vi "CRYInsert All.vi"(4 "Waves":T1 {"Y dB ref" format="%.1f"; "Y axis" items=["Log", "Lin"]; "Y data" items=["dB", "Lin"]; "X data" items=["dB", "Lin"]}, 6 "Results":T3 {"Margin" format="%.2f"}, 7 "sOption2":string, 8 "sOption1":string, 9 "Curves":T5 {"Z data" items=["dB", "Lin"]; "X data" items=["dB", "Lin"]; "Y data" items=["dB", "Lin"]; "Z dB ref" format="%.1f"; "Z axis" items=["Log", "Lin"]; "X dB ref" format="%.1f"; "X axis" items=["Log", "Lin"]; "Y axis" items=["Log", "Lin"]; "Y dB ref" format="%.1f"; "Curve"."z" format="%.2f"; "Curve"."y" format="%.2f"; "Curve"."x" format="%.2f"}, 10 "Step No.":i32, 11 "Type In":enum16{"Curves", "Values", "Results", "WFM"}(ring)) -> (2 "Inserted Names Out":string[](array[string]), 3 "Type Out":enum16{"Curves", "Values", "Results", "WFM"}(ring))   [LabVIEW 2013]
uses:
  CRYSystem/Typedef Control/CRYData Cluster Array.ctl
  CRYSystem/Typedef Control/CRYData Cluster.ctl
  CRYSystem/Typedef Control/CRYResult Cluster Array.ctl
  CRYSystem/Typedef Control/CRYResult Cluster.ctl
  CRYSystem/Typedef Control/CRYWaveform Cluster Array.ctl
  CRYSystem/Typedef Control/CRYWaveform Cluster.ctl
  Global/CRYCurve Library Global.vi
  CRYSystem/Task Sequence/CRYProject Run Control Global.vi
panel:
  out "wav2":i32[](array[numeric])
  out "wav1":i32[](array[numeric])
  out "res2":i32[](array[numeric])
  out "res1":i32[](array[numeric])
  out "val1":i32[](array[numeric])
  out "val2":i32[](array[numeric])
  out "cur1":i32[](array[numeric])
  out "cur2":i32[](array[numeric])
  out "x-y":i32[](array[numeric])
  out "Type":string[](array[string])
  out "Deleted Names":string[](array[string])
  out "Inserted Names":string[](array[string])
  out "Inserted Index":i32[](array[numeric])
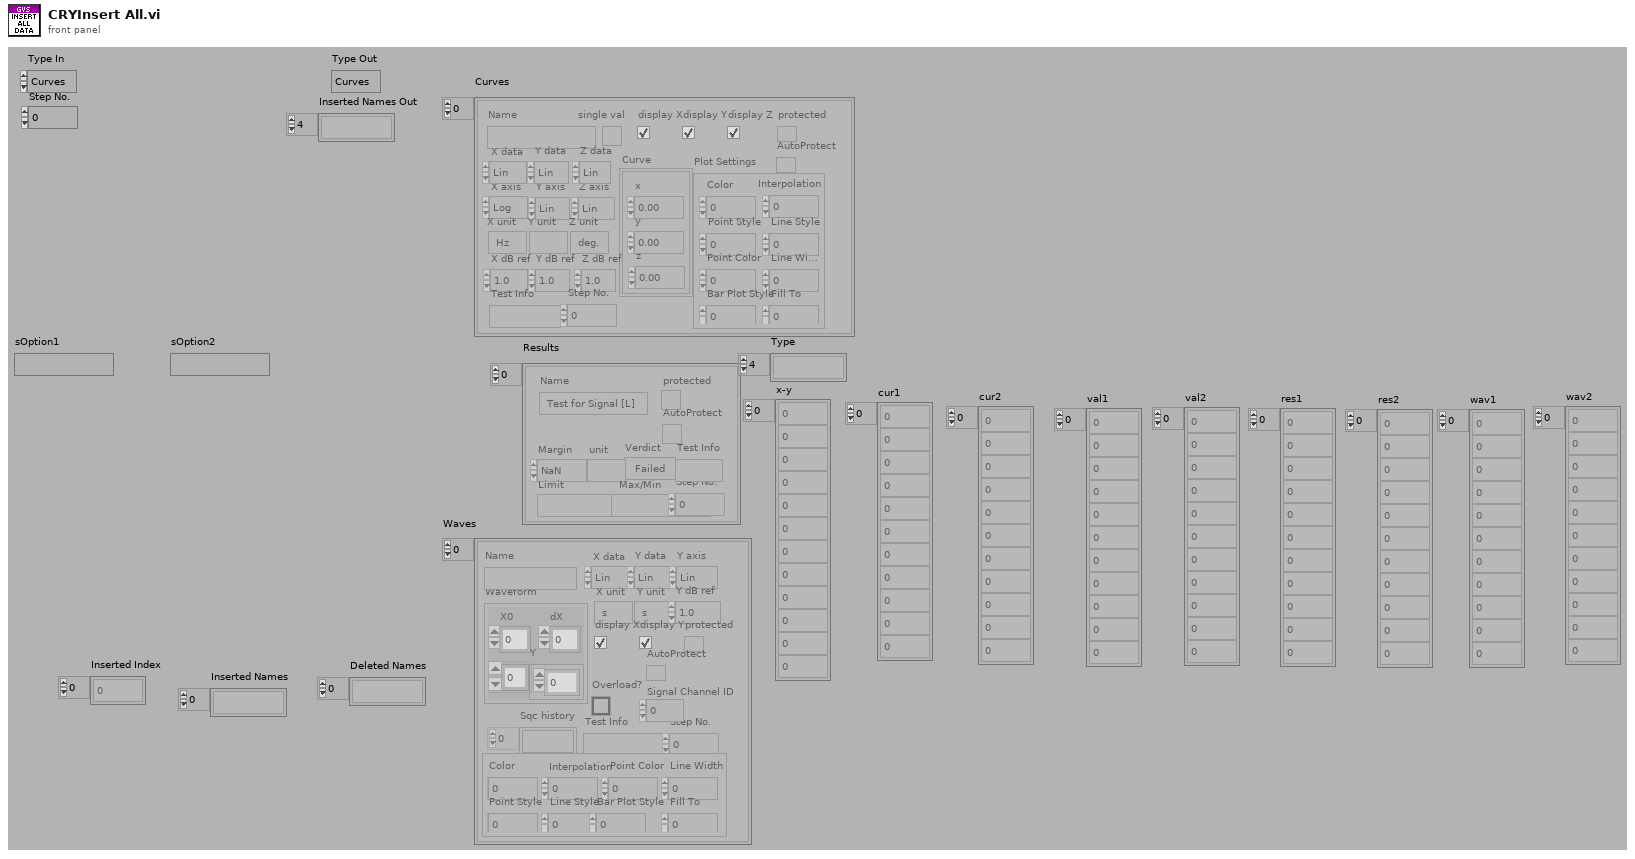
[diagram p1: front panel]
types:
  T1 = typedef "CRYWaveform Cluster Array.ctl" = T2[]
  T2 = typedef "CRYWaveform Cluster.ctl" = cluster{"Waveform":cluster{"X0":dbl, "dX":dbl, "Y":sgl[]}, "X data":u16, "Y data":u16, "Y axis":u16, "X unit":string, "Y unit":string, "Y dB ref":dbl, "display Y":bool, "display X":bool, "Overload?":bool, "Test Info":string, "Step No.":i32, "Name":string, "protected":bool, "Sqc history":string[], "Signal Channel ID":i32, "Plot Settings":cluster{"Color":u32, "Interpolation":u8, "Point Style":u8, "Line Style":u8, "Point Color":u32, "Line Width":u8, "Bar Plot Style":u8, "Fill To":i16}, "AutoProtect":bool}
  T3 = typedef "CRYResult Cluster Array.ctl" = T4[]
  T4 = typedef "CRYResult Cluster.ctl" = cluster{"Name":string, "Margin":dbl, "unit":string, "Verdict":bool, "Limit":string, "Max/Min":string, "protected":bool, "Step No.":i32, "Test Info":string, "AutoProtect":bool}
  T5 = typedef "CRYData Cluster Array.ctl" = T6[]
  T6 = typedef "CRYData Cluster.ctl" = cluster{"Name":string, "Curve":cluster{"x":dbl, "y":dbl, "z":dbl}[], "X data":u16, "Y data":u16, "Z data":u16, "X axis":u16, "Y axis":u16, "Z axis":u16, "X unit":string, "Y unit":string, "Z unit":string, "X dB ref":dbl, "Y dB ref":dbl, "Z dB ref":dbl, "single val":bool, "protected":bool, "display X":bool, "display Y":bool, "display Z":bool, "Test Info":string, "Step No.":i32, "Plot Settings":cluster{"Color":u32, "Interpolation":u8, "Point Style":u8, "Line Style":u8, "Point Color":u32, "Line Width":u8, "Bar Plot Style":u8, "Fill To":i16}, "AutoProtect":bool}
  T7 = cluster{"Color":u32, "Interpolation":u8, "Point Style":u8, "Line Style":u8, "Point Color":u32, "Line Width":u8, "Bar Plot Style":u8, "Fill To":i16}
  T8 = cluster{"CurveOld":string[], "ValueOld":string[], "ResultOld":string[], "WFMOld":string[], "CurveNew":string[], "ValueNew":string[], "ResultNew":string[], "WFMNew":string[]}
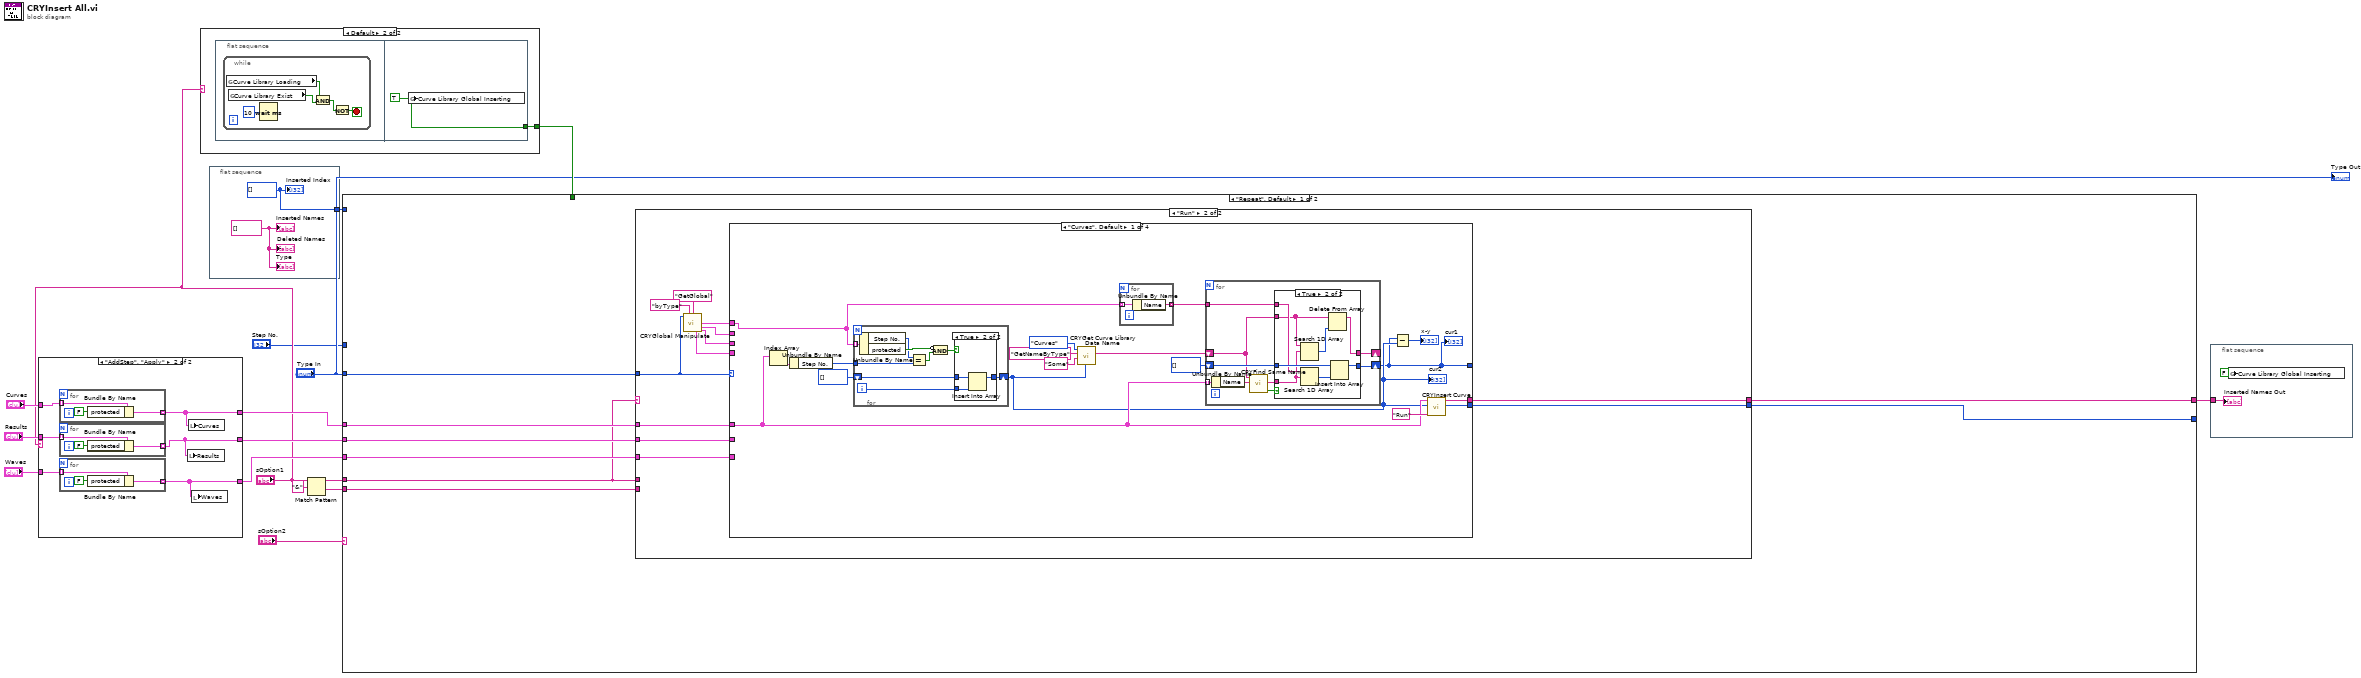
[diagram p0: block diagram]
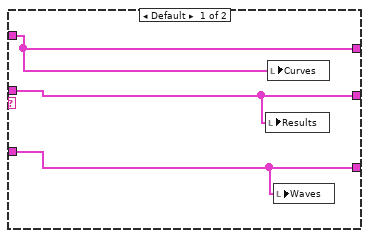
[diagram p2: hidden frame]
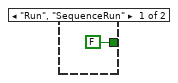
[diagram p3: hidden frame]
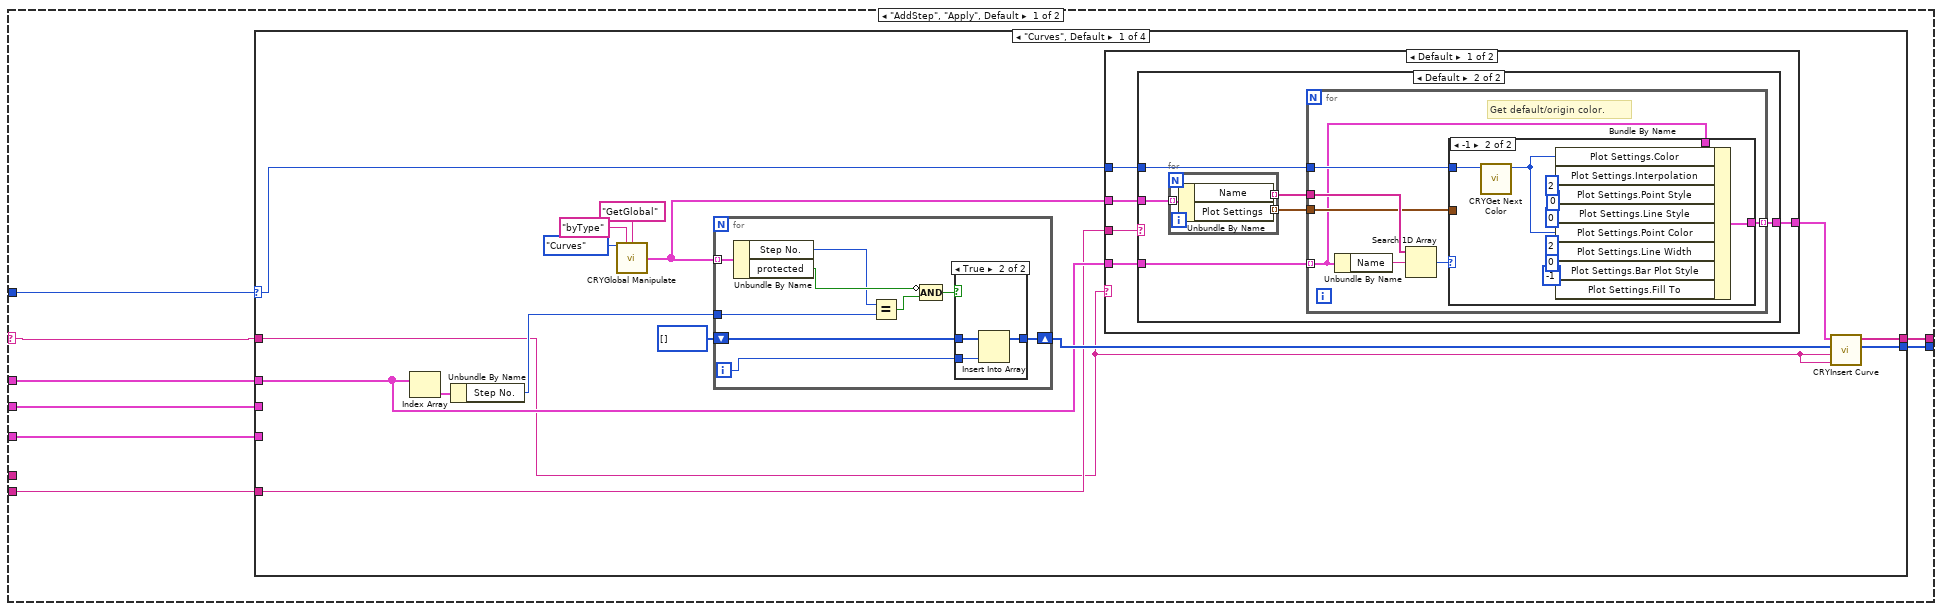
[diagram p4: hidden frame]
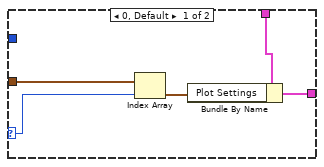
[diagram p7: hidden frame]
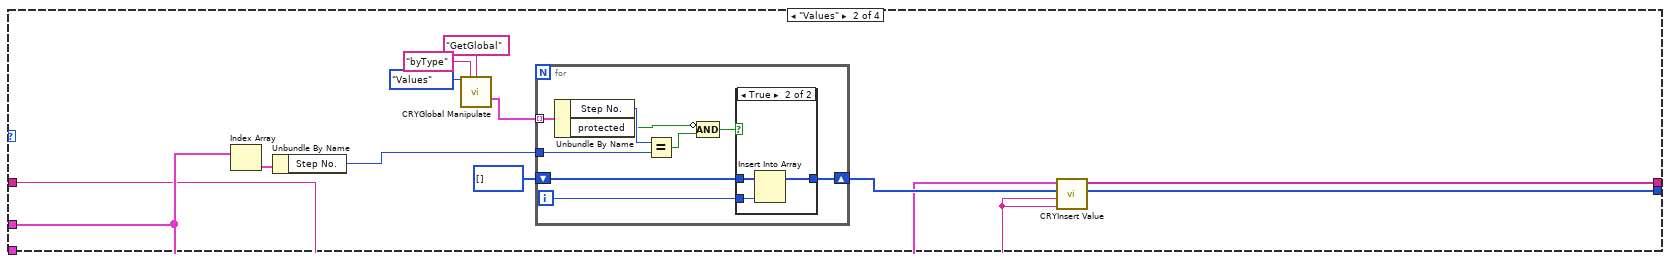
[diagram p9: hidden frame]
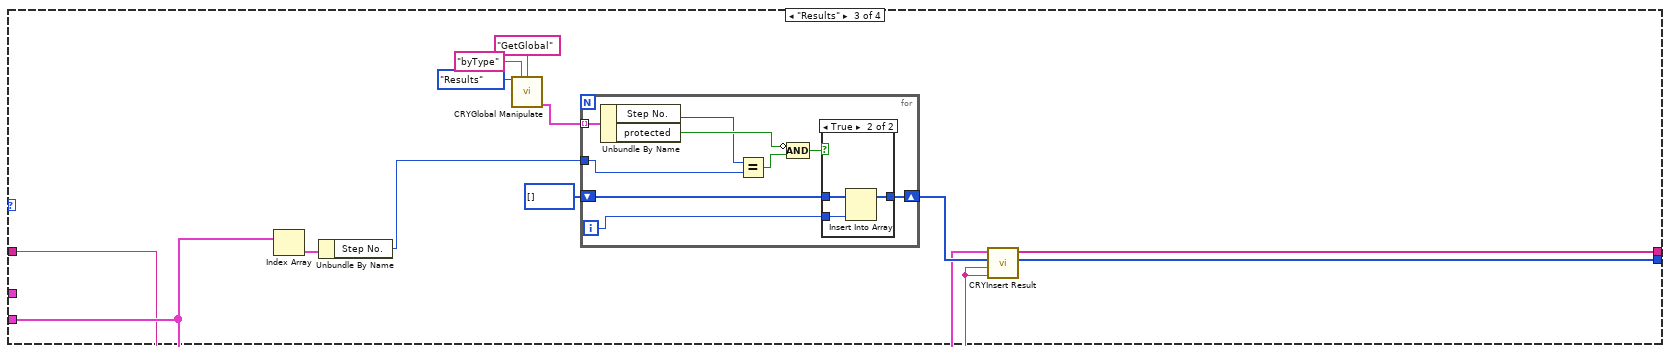
[diagram p11: hidden frame]
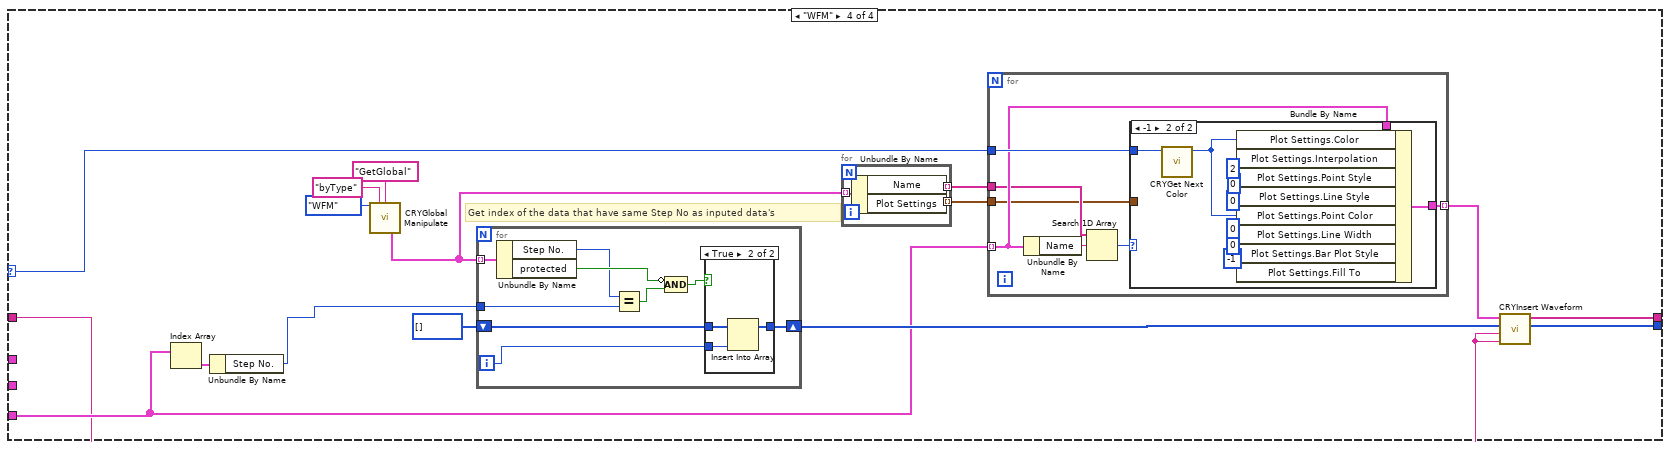
[diagram p13: hidden frame]
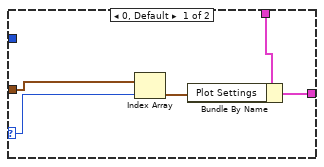
[diagram p14: hidden frame]
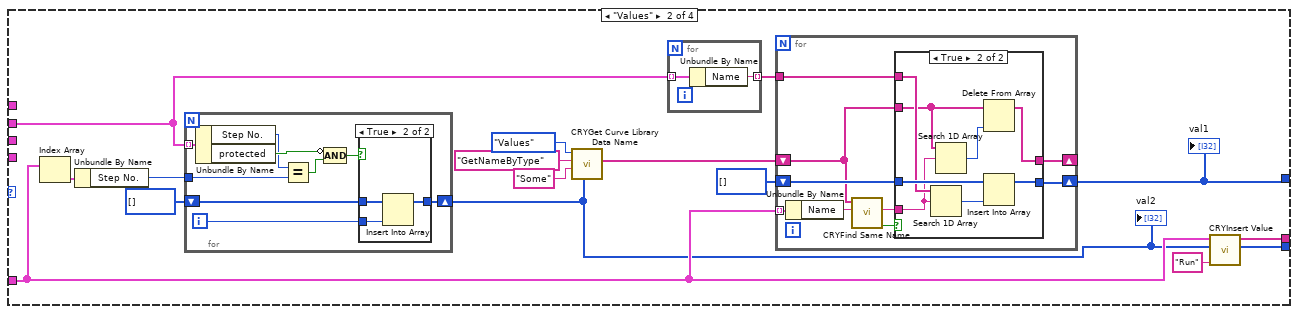
[diagram p18: hidden frame]
diagram:
  n1 = case shown="\"AddStep\", \"Apply\"" "sOption1" {
    tunnel: "Curves" -> [w19 w25]
    tunnel: [w19 w24] -> w7
    tunnel: "Waves" -> [w18 w23]
    tunnel: [w18 w22] -> w5
    tunnel: "Results" -> [w17 w21]
    tunnel: [w17 w20] -> w3
    frame Default {
      n2 = local write "Results"(w17) -> ()
      n3 = local write "Curves"(w19) -> ()
      n4 = local write "Waves"(w18) -> ()
    }
    frame "AddStep", "Apply" {
      n5 = for {
        tunnel: w25 -> [w34] mode=indexing
        tunnel: [w32] -> w24 mode=indexing
        n6 = Bundle By Name(cluster=w34, "protected"=FALSE) -> (w32:T6)
      }
      n7 = for {
        tunnel: w21 -> [w31] mode=indexing
        tunnel: [w29] -> w20 mode=indexing
        n8 = Bundle By Name(cluster=w31, "protected"=FALSE) -> (w29:T4)
      }
      n9 = for {
        tunnel: w23 -> [w28] mode=indexing
        tunnel: [w26] -> w22 mode=indexing
        n10 = Bundle By Name(cluster=w28, "protected"=FALSE) -> (w26:T2)
      }
      n11 = local write "Results"(w20) -> ()
      n12 = local write "Curves"(w24) -> ()
      n13 = local write "Waves"(w22) -> ()
    }
  }
  n14 = case shown="Default" "sOption1" {
    tunnel: [FALSE ("Curve Library Global Inserting") w36] -> w16
    frame "Run", "SequenceRun" {
    }
    frame Default {
      n15 = flat-sequence {
        tunnel: [w42] -> w36
        frame #0 {
          n16 = while {
            stop <- w37 stop-if-true
            n17 = global read "CRYCurve Library Global.vi" "Curve Library Loading"() -> (w39:bool)
            n18 = global read "CRYCurve Library Global.vi" "Curve Library Exist"() -> (w38:bool)
            n19 = Wait (ms)(milliseconds to wait=u32 10) -> ()  [unwired: 1 out]
            n20 = And(x=w39, y=w38) -> (x .and. y?=w40:bool)
            n21 = Not(x=w40) -> (.not. x?=w37:bool)
          }
        }
        frame #1 {
          w42 = TRUE ("Curve Library Global Inserting")
          n22 = global write "CRYCurve Library Global.vi" "Curve Library Global Inserting"(w42) -> ()
        }
      }
    }
  }
  n23 = flat-sequence {
    tunnel: [w44] -> w9
    frame #0 {
      w43 = string[] [] ("Inserted Names")
      w44 = i32[] [] ("Index")
      "Inserted Index" <- w44
      "Inserted Names" <- w43
      "Deleted Names" <- w43
      "Type" <- w43
    }
  }
  n24 = Match Pattern(string="sOption1", regular expression="&") -> (before substring=w13:string, after substring=w12:string)  [unwired: 1 in, 2 out]
  n25 = case shown="\"Repeat\", Default" "sOption2" {
    tunnel: w16 -> [_ _]
    tunnel: [w46 w464] -> w15
    tunnel: [w52 w461] -> _
    tunnel: w7 -> [w49 w465]
    tunnel: "Type In" -> [w45 w463]
    tunnel: w13 -> [w47 _]
    tunnel: w12 -> [w48 _]
    tunnel: w9 -> [_ _]
    tunnel: w3 -> [w51 w453]
    tunnel: w5 -> [w50 w452]
    tunnel: "Step No." -> [_ w444]
    frame "Repeat", Default {
      n26 = case shown="\"Run\"" w47 {
        selector: w47 -> [w53 _]
        tunnel: [w60 w242] -> w46
        tunnel: [w59 w241] -> w52
        tunnel: w45 -> [w54 w235]
        tunnel: w51 -> [w58 w240]
        tunnel: w50 -> [w57 w239]
        tunnel: w49 -> [w56 w238]
        tunnel: w48 -> [w55 _]
        tunnel: w47 -> [_ _]
        frame "AddStep", "Apply", Default {
          n27 = case shown="\"Curves\", Default" w54 {
            selector: w54 -> [w66 _ _ w182]
            tunnel: w56 -> [w73 w135 _ _]
            tunnel: [w75 w138 w163 w192] -> w60
            tunnel: [w71 w136 w160 w188] -> w59
            tunnel: w55 -> [w70 _ _ _]
            tunnel: w58 -> [_ _ w161 _]
            tunnel: w57 -> [_ _ _ w190]
            tunnel: w53 -> [w61 w127 w152 w177]
            frame "Curves", Default {
              n28 = Index Array(array=w73) -> (element=w67:T6)  [unwired: 1 in]
              n29 = Unbundle By Name(w67) -> ("Step No."=w68:i32)
              n30 = call "CRYGlobal Manipulate.vi"("Type"=enum16{"Curves", "Values", "Results", "WFM"}."Curves", "sOption"="byType", "sAction"="GetGlobal") -> ("Curves Out"=w62:T6[])  [unwired: 6 in, 6 out]
              n31 = for {
                tunnel: w68 -> [w76]
                tunnel: w62 -> [w82] mode=indexing
                shift-right: [w83] -> w74
                shift-left: i32[] [] ("Index") -> [w84]
                i -> [w81]
                n32 = Unbundle By Name(w82) -> ("Step No."=w77:i32, "protected"=w78:bool)
                n33 = Equal?(x=w77, y=w76) -> (x = y?=w80:bool)
                n34 = Compound Arithmetic op=AND(invert w78, w80) -> (w79:bool)
                n35 = case shown="True" w79 {
                  tunnel: [w85 w87] -> w83
                  tunnel: w84 -> [w85 w88]
                  tunnel: w81 -> [_ w86]
                  frame False {
                  }
                  frame True {
                    n36 = Insert Into Array(array=w88, new element=w86) -> (w87:i32[])  [unwired: 1 in]
                  }
                }
              }
              n37 = case shown="Default" w61 {
                tunnel: w66 -> [w93 _]
                tunnel: w73 -> [w92 w126]
                tunnel: [w91 w126] -> w72
                tunnel: w70 -> [w90 _]
                tunnel: w62 -> [w89 _]
                frame Default {
                  n38 = case shown="Default" w90 {
                    tunnel: w93 -> [_ w100]
                    tunnel: w92 -> [w94 w99]
                    tunnel: [w94 w98] -> w91
                    tunnel: w89 -> [_ w97]
                    frame "UsePlot" {
                    }
                    frame Default {
                      n39 = for {
                        tunnel: w97 -> [w103] mode=indexing
                        tunnel: [w102] -> w96 mode=indexing
                        tunnel: [w101] -> w95 mode=indexing
                        n40 = Unbundle By Name(w103) -> ("Name"=w102:string, "Plot Settings"=w101:T7)
                      }
                      n41 = for {
                        tunnel: w99 -> [w104] mode=indexing
                        tunnel: [w109] -> w98 mode=indexing
                        tunnel: w100 -> [w110]
                        tunnel: w96 -> [w108]
                        tunnel: w95 -> [w105]
                        # "Get default/origin color."
                        n42 = Unbundle By Name(w104) -> ("Name"=w107:string)
                        n43 = Search 1D Array(1D array=w108, element=w107) -> (index of element=w106:i32)  [unwired: 1 out]
                        n44 = case shown="-1" w106 {
                          selector: w106 -> [w112 _]
                          tunnel: w110 -> [_ w125]
                          tunnel: [w114 w124] -> w109
                          tunnel: w104 -> [w115 w123]
                          tunnel: w105 -> [w113 _]
                          frame 0, Default {
                            n45 = Index Array(array=w113, index=w112) -> (element=w111:T7)
                            n46 = Bundle By Name(cluster=w115, "Plot Settings"=w111) -> (w114:T6)
                          }
                          frame -1 {
                            n47 = call "CRYGet Next Color.vi"("Type"=w125) -> ("Color"=w119:u32)  [unwired: 10 out]
                            n48 = Bundle By Name(cluster=w123, "Plot Settings.Color"=w119, "Plot Settings.Interpolation"=u8 2, "Plot Settings.Point Style"=u8 0, "Plot Settings.Line Style"=u8 0, "Plot Settings.Point Color"=w119, "Plot Settings.Line Width"=u8 2, "Plot Settings.Bar Plot Style"=u8 0, "Plot Settings.Fill To"=i16 -1) -> (w124:T6)
                          }
                        }
                      }
                    }
                  }
                }
                frame "Protect_Setting" {
                }
              }
              n49 = call "CRYInsert Curve.vi"("sOptionUpdate"=w61, "sOption"=w61, "Index"=w74, "Curve"=w72) -> ("Inserted Index"=w71:i32[], "Inserted Name Out"=w75:string[])  [unwired: 1 in, 5 out]
            }
            frame "Values" {
              n50 = Index Array(array=w135) -> (element=w132:T6)  [unwired: 1 in]
              n51 = Unbundle By Name(w132) -> ("Step No."=w133:i32)
              n52 = call "CRYGlobal Manipulate.vi"("Type"=enum16{"Curves", "Values", "Results", "WFM"}."Values", "sOption"="byType", "sAction"="GetGlobal") -> ("Values Out"=w128:T6[])  [unwired: 6 in, 6 out]
              n53 = for {
                tunnel: w133 -> [w139]
                tunnel: w128 -> [w145] mode=indexing
                shift-right: [w146] -> w137
                shift-left: i32[] [] ("Index") -> [w147]
                i -> [w144]
                n54 = Unbundle By Name(w145) -> ("Step No."=w141:i32, "protected"=w140:bool)
                n55 = Equal?(x=w141, y=w139) -> (x = y?=w143:bool)
                n56 = Compound Arithmetic op=AND(invert w140, w143) -> (w142:bool)
                n57 = case shown="True" w142 {
                  tunnel: [w148 w150] -> w146
                  tunnel: w147 -> [w148 w151]
                  tunnel: w144 -> [_ w149]
                  frame False {
                  }
                  frame True {
                    n58 = Insert Into Array(array=w151, new element=w149) -> (w150:i32[])  [unwired: 1 in]
                  }
                }
              }
              n59 = call "CRYInsert Value.vi"("sOptionUpdate"=w127, "sOption"=w127, "Index"=w137, "Value"=w135) -> ("Inserted Index"=w136:i32[], "Inserted Name Out"=w138:string[])  [unwired: 6 out]
            }
            frame "Results" {
              n60 = Index Array(array=w161) -> (element=w157:T4)  [unwired: 1 in]
              n61 = Unbundle By Name(w157) -> ("Step No."=w158:i32)
              n62 = call "CRYGlobal Manipulate.vi"("Type"=enum16{"Curves", "Values", "Results", "WFM"}."Results", "sOption"="byType", "sAction"="GetGlobal") -> ("Results Out"=w153:T4[])  [unwired: 6 in, 6 out]
              n63 = for {
                tunnel: w158 -> [w164]
                tunnel: w153 -> [w170] mode=indexing
                shift-right: [w171] -> w162
                shift-left: i32[] [] ("Index") -> [w172]
                i -> [w169]
                n64 = Unbundle By Name(w170) -> ("Step No."=w165:i32, "protected"=w166:bool)
                n65 = Equal?(x=w165, y=w164) -> (x = y?=w168:bool)
                n66 = Compound Arithmetic op=AND(invert w166, w168) -> (w167:bool)
                n67 = case shown="True" w167 {
                  tunnel: [w173 w175] -> w171
                  tunnel: w172 -> [w173 w176]
                  tunnel: w169 -> [_ w174]
                  frame False {
                  }
                  frame True {
                    n68 = Insert Into Array(array=w176, new element=w174) -> (w175:i32[])  [unwired: 1 in]
                  }
                }
              }
              n69 = call "CRYInsert Result.vi"("sOptionUpdate"=w152, "sOption"=w152, "Index"=w162, "Result"=w161) -> ("Inserted Index"=w160:i32[], "Inserted Name Out"=w163:string[])  [unwired: 6 out]
            }
            frame "WFM" {
              # "Get index of the data that have same Step No as inputed data's"
              n70 = Index Array(array=w190) -> (element=w185:T2)  [unwired: 1 in]
              n71 = Unbundle By Name(w185) -> ("Step No."=w186:i32)
              n72 = call "CRYGlobal Manipulate.vi"("Type"=enum16{"Curves", "Values", "Results", "WFM"}."WFM", "sOption"="byType", "sAction"="GetGlobal") -> ("WFM Out"=w178:T2[])  [unwired: 6 in, 6 out]
              n73 = for {
                tunnel: w186 -> [w222]
                tunnel: w178 -> [w224] mode=indexing
                shift-right: [w225] -> w191
                shift-left: i32[] [] ("Index") -> [w226]
                i -> [w218]
                n74 = Unbundle By Name(w224) -> ("Step No."=w219:i32, "protected"=w221:bool)
                n75 = Equal?(x=w219, y=w222) -> (x = y?=w220:bool)
                n76 = Compound Arithmetic op=AND(invert w221, w220) -> (w223:bool)
                n77 = case shown="True" w223 {
                  tunnel: [w227 w229] -> w225
                  tunnel: w226 -> [w227 w230]
                  tunnel: w218 -> [_ w228]
                  frame False {
                  }
                  frame True {
                    n78 = Insert Into Array(array=w230, new element=w228) -> (w229:i32[])  [unwired: 1 in]
                  }
                }
              }
              n79 = for {
                tunnel: w178 -> [w195] mode=indexing
                tunnel: [w194] -> w184 mode=indexing
                tunnel: [w193] -> w183 mode=indexing
                n80 = Unbundle By Name(w195) -> ("Name"=w194:string, "Plot Settings"=w193:T7)
              }
              n81 = for {
                tunnel: w190 -> [w198] mode=indexing
                tunnel: [w201] -> w189 mode=indexing
                tunnel: w182 -> [w202]
                tunnel: w184 -> [w197]
                tunnel: w183 -> [w196]
                n82 = Unbundle By Name(w198) -> ("Name"=w200:string)
                n83 = Search 1D Array(1D array=w197, element=w200) -> (index of element=w199:i32)  [unwired: 1 out]
                n84 = case shown="-1" w199 {
                  selector: w199 -> [w205 _]
                  tunnel: w202 -> [_ w217]
                  tunnel: [w206 w216] -> w201
                  tunnel: w198 -> [w207 w215]
                  tunnel: w196 -> [w203 _]
                  frame 0, Default {
                    n85 = Index Array(array=w203, index=w205) -> (element=w204:T7)
                    n86 = Bundle By Name(cluster=w207, "Plot Settings"=w204) -> (w206:T2)
                  }
                  frame -1 {
                    n87 = call "CRYGet Next Color.vi"("Type"=w217) -> ("Color"=w211:u32)  [unwired: 10 out]
                    n88 = Bundle By Name(cluster=w215, "Plot Settings.Color"=w211, "Plot Settings.Interpolation"=u8 2, "Plot Settings.Point Style"=u8 0, "Plot Settings.Line Style"=u8 0, "Plot Settings.Point Color"=w211, "Plot Settings.Line Width"=u8 0, "Plot Settings.Bar Plot Style"=u8 0, "Plot Settings.Fill To"=i16 -1) -> (w216:T2)
                  }
                }
              }
              n89 = call "CRYInsert Waveform.vi"("sOptionUpdate"=w177, "sOption"=w177, "Index"=w191, "Waveform"=w189) -> ("Inserted Index"=w188:i32[], "Inserted Name Out"=w192:string[])  [unwired: 6 out]
            }
          }
        }
        frame "Run" {
          n90 = call "CRYGlobal Manipulate.vi"("Type"=w235, "sOption"="byType", "sAction"="GetGlobal") -> ("Curves Out"=w234:T6[], "Values Out"=w233:T6[], "WFM Out"=w231:T2[], "Results Out"=w232:T4[])  [unwired: 6 in, 3 out]
          n91 = case shown="\"Curves\", Default" w235 {
            tunnel: w238 -> [w249 w299 _ _]
            tunnel: [w259 w309 w359 w409] -> w242
            tunnel: [w258 w308 w358 w408] -> w241
            tunnel: w240 -> [_ _ w349 _]
            tunnel: w239 -> [_ _ _ w399]
            tunnel: w234 -> [w248 _ _ _]
            tunnel: w233 -> [_ w298 _ _]
            tunnel: w232 -> [_ _ w348 _]
            tunnel: w231 -> [_ _ _ w398]
            tunnel: [w244 w295 _ _] -> _
            frame "Curves", Default {
              n92 = Index Array(array=w249) -> (element=w256:T6)  [unwired: 1 in]
              n93 = Unbundle By Name(w256) -> ("Step No."=w254:i32)
              n94 = for {
                tunnel: w254 -> [w281]
                tunnel: w248 -> [w287] mode=indexing
                shift-right: [w288] -> w245
                shift-left: i32[] [] ("Index") -> [w289]
                i -> [w286]
                n95 = Unbundle By Name(w287) -> ("Step No."=w282:i32, "protected"=w283:bool)
                n96 = Equal?(x=w282, y=w281) -> (x = y?=w285:bool)
                n97 = Compound Arithmetic op=AND(invert w283, w285) -> (w284:bool)
                n98 = case shown="True" w284 {
                  tunnel: [w290 w292] -> w288
                  tunnel: w289 -> [w290 w293]
                  tunnel: w286 -> [_ w291]
                  frame False {
                  }
                  frame True {
                    n99 = Insert Into Array(array=w293, new element=w291) -> (w292:i32[])  [unwired: 1 in]
                  }
                }
              }
              "cur2" <- w245
              n100 = call "CRYGet Curve Library Data Name.vi"("nData"=w245, "sOption"="Some", "sAction"="GetNameByType", "Type"=enum16{"Curves", "Values", "Results", "WFM"}."Curves") -> ("sNames"=w250:string[])  [unwired: 4 in, 3 out]
              n101 = for {
                tunnel: w248 -> [w280] mode=indexing
                tunnel: [w279] -> w246 mode=indexing
                n102 = Unbundle By Name(w280) -> ("Name"=w279:string)
              }
              n103 = for {
                tunnel: w249 -> [w268] mode=indexing
                shift-right: [w264] -> w244
                shift-left: i32[] [] -> [w265]
                tunnel: w246 -> [w262]
                shift-right: [w260] -> _
                shift-left: w250 -> [w261]
                n104 = Unbundle By Name(w268) -> ("Name"=w267:string)
                n105 = call "CRYFind Same Name.vi"("Name"=w267, "sNames"=w261) -> ("bResult"=w266:bool, "NameOut"=w263:string)  [unwired: 7 in, 1 out]
                n106 = case shown="True" w266 {
                  tunnel: w265 -> [w270 w278]
                  tunnel: [w270 w277] -> w264
                  tunnel: w263 -> [_ w272]
                  tunnel: w262 -> [_ w276]
                  tunnel: w261 -> [w269 w273]
                  tunnel: [w269 w274] -> w260
                  frame False {
                  }
                  frame True {
                    n107 = Search 1D Array(1D array=w276, element=w272) -> (index of element=w275:i32)  [unwired: 1 in]
                    n108 = Search 1D Array(1D array=w273, element=w272) -> (index of element=w271:i32)  [unwired: 1 in]
                    n109 = Delete From Array(array=w273, index=w271) -> (array with subset deleted=w274:string[])  [unwired: 1 in, 1 out]
                    n110 = Insert Into Array(array=w278, new element=w275) -> (w277:i32[])  [unwired: 1 in]
                  }
                }
              }
              "cur1" <- w244
              n111 = Subtract(x=w244, y=w245) -> (x-y=→"x-y":i32[])
              n112 = call "CRYInsert Curve.vi"("sOptionUpdate"="Run", "Index"=w245, "Curve"=w249) -> ("Inserted Index"=w258:i32[], "Inserted Name Out"=w259:string[])  [unwired: 2 in, 5 out]
            }
            frame "Values" {
              n113 = Index Array(array=w299) -> (element=w306:T6)  [unwired: 1 in]
              n114 = Unbundle By Name(w306) -> ("Step No."=w304:i32)
              n115 = for {
                tunnel: w304 -> [w331]
                tunnel: w298 -> [w337] mode=indexing
                shift-right: [w338] -> w294
                shift-left: i32[] [] ("Index") -> [w339]
                i -> [w336]
                n116 = Unbundle By Name(w337) -> ("Step No."=w332:i32, "protected"=w333:bool)
                n117 = Equal?(x=w332, y=w331) -> (x = y?=w335:bool)
                n118 = Compound Arithmetic op=AND(invert w333, w335) -> (w334:bool)
                n119 = case shown="True" w334 {
                  tunnel: [w340 w342] -> w338
                  tunnel: w339 -> [w340 w343]
                  tunnel: w336 -> [_ w341]
                  frame False {
                  }
                  frame True {
                    n120 = Insert Into Array(array=w343, new element=w341) -> (w342:i32[])  [unwired: 1 in]
                  }
                }
              }
              "val2" <- w294
              n121 = call "CRYGet Curve Library Data Name.vi"("nData"=w294, "sOption"="Some", "sAction"="GetNameByType", "Type"=enum16{"Curves", "Values", "Results", "WFM"}."Values") -> ("sNames"=w300:string[])  [unwired: 4 in, 3 out]
              n122 = for {
                tunnel: w298 -> [w330] mode=indexing
                tunnel: [w329] -> w296 mode=indexing
                n123 = Unbundle By Name(w330) -> ("Name"=w329:string)
              }
              n124 = for {
                tunnel: w299 -> [w318] mode=indexing
                shift-right: [w314] -> w295
                shift-left: i32[] [] -> [w315]
                tunnel: w296 -> [w312]
                shift-right: [w310] -> _
                shift-left: w300 -> [w311]
                n125 = Unbundle By Name(w318) -> ("Name"=w317:string)
                n126 = call "CRYFind Same Name.vi"("Name"=w317, "sNames"=w311) -> ("bResult"=w316:bool, "NameOut"=w313:string)  [unwired: 7 in, 1 out]
                n127 = case shown="True" w316 {
                  tunnel: w315 -> [w320 w328]
                  tunnel: [w320 w327] -> w314
                  tunnel: w313 -> [_ w322]
                  tunnel: w312 -> [_ w326]
                  tunnel: w311 -> [w319 w323]
                  tunnel: [w319 w324] -> w310
                  frame False {
                  }
                  frame True {
                    n128 = Search 1D Array(1D array=w326, element=w322) -> (index of element=w325:i32)  [unwired: 1 in]
                    n129 = Search 1D Array(1D array=w323, element=w322) -> (index of element=w321:i32)  [unwired: 1 in]
                    n130 = Delete From Array(array=w323, index=w321) -> (array with subset deleted=w324:string[])  [unwired: 1 in, 1 out]
                    n131 = Insert Into Array(array=w328, new element=w325) -> (w327:i32[])  [unwired: 1 in]
                  }
                }
              }
              "val1" <- w295
              n132 = call "CRYInsert Value.vi"("sOptionUpdate"="Run", "Index"=w294, "Value"=w299) -> ("Inserted Index"=w308:i32[], "Inserted Name Out"=w309:string[])  [unwired: 1 in, 6 out]
            }
            frame "Results" {
              n133 = Index Array(array=w349) -> (element=w356:T4)  [unwired: 1 in]
              n134 = Unbundle By Name(w356) -> ("Step No."=w354:i32)
              n135 = for {
                tunnel: w354 -> [w381]
                tunnel: w348 -> [w387] mode=indexing
                shift-right: [w388] -> w344
                shift-left: i32[] [] ("Index") -> [w389]
                i -> [w386]
                n136 = Unbundle By Name(w387) -> ("Step No."=w382:i32, "protected"=w383:bool)
                n137 = Equal?(x=w382, y=w381) -> (x = y?=w385:bool)
                n138 = Compound Arithmetic op=AND(invert w383, w385) -> (w384:bool)
                n139 = case shown="True" w384 {
                  tunnel: [w390 w392] -> w388
                  tunnel: w389 -> [w390 w393]
                  tunnel: w386 -> [_ w391]
                  frame False {
                  }
                  frame True {
                    n140 = Insert Into Array(array=w393, new element=w391) -> (w392:i32[])  [unwired: 1 in]
                  }
                }
              }
              "res2" <- w344
              n141 = call "CRYGet Curve Library Data Name.vi"("nData"=w344, "sOption"="Some", "sAction"="GetNameByType", "Type"=enum16{"Curves", "Values", "Results", "WFM"}."Results") -> ("sNames"=w350:string[])  [unwired: 4 in, 3 out]
              n142 = for {
                tunnel: w348 -> [w380] mode=indexing
                tunnel: [w379] -> w346 mode=indexing
                n143 = Unbundle By Name(w380) -> ("Name"=w379:string)
              }
              n144 = for {
                tunnel: w349 -> [w368] mode=indexing
                shift-right: [w364] -> w345
                shift-left: i32[] [] -> [w365]
                tunnel: w346 -> [w362]
                shift-right: [w360] -> _
                shift-left: w350 -> [w361]
                n145 = Unbundle By Name(w368) -> ("Name"=w367:string)
                n146 = call "CRYFind Same Name.vi"("Name"=w367, "sNames"=w361) -> ("bResult"=w366:bool, "NameOut"=w363:string)  [unwired: 7 in, 1 out]
                n147 = case shown="True" w366 {
                  tunnel: w365 -> [w370 w378]
                  tunnel: [w370 w377] -> w364
                  tunnel: w363 -> [_ w372]
                  tunnel: w362 -> [_ w376]
                  tunnel: w361 -> [w369 w373]
                  tunnel: [w369 w374] -> w360
                  frame False {
                  }
                  frame True {
                    n148 = Search 1D Array(1D array=w373, element=w372) -> (index of element=w371:i32)  [unwired: 1 in]
                    n149 = Search 1D Array(1D array=w376, element=w372) -> (index of element=w375:i32)  [unwired: 1 in]
                    n150 = Delete From Array(array=w373, index=w371) -> (array with subset deleted=w374:string[])  [unwired: 1 in, 1 out]
                    n151 = Insert Into Array(array=w378, new element=w375) -> (w377:i32[])  [unwired: 1 in]
                  }
                }
              }
              "res1" <- w345
              n152 = call "CRYInsert Result.vi"("sOptionUpdate"="Run", "Index"=w344, "Result"=w349) -> ("Inserted Index"=w358:i32[], "Inserted Name Out"=w359:string[])  [unwired: 1 in, 6 out]
            }
            frame "WFM" {
              n153 = Index Array(array=w399) -> (element=w406:T2)  [unwired: 1 in]
              n154 = Unbundle By Name(w406) -> ("Step No."=w404:i32)
              n155 = for {
                tunnel: w404 -> [w431]
                tunnel: w398 -> [w437] mode=indexing
                shift-right: [w438] -> w394
                shift-left: i32[] [] ("Index") -> [w439]
                i -> [w436]
                n156 = Unbundle By Name(w437) -> ("Step No."=w432:i32, "protected"=w433:bool)
                n157 = Equal?(x=w432, y=w431) -> (x = y?=w435:bool)
                n158 = Compound Arithmetic op=AND(invert w433, w435) -> (w434:bool)
                n159 = case shown="True" w434 {
                  tunnel: [w440 w442] -> w438
                  tunnel: w439 -> [w440 w443]
                  tunnel: w436 -> [_ w441]
                  frame False {
                  }
                  frame True {
                    n160 = Insert Into Array(array=w443, new element=w441) -> (w442:i32[])  [unwired: 1 in]
                  }
                }
              }
              "wav2" <- w394
              n161 = call "CRYGet Curve Library Data Name.vi"("nData"=w394, "sOption"="Some", "sAction"="GetNameByType", "Type"=enum16{"Curves", "Values", "Results", "WFM"}."WFM") -> ("sNames"=w400:string[])  [unwired: 4 in, 3 out]
              n162 = for {
                tunnel: w398 -> [w430] mode=indexing
                tunnel: [w429] -> w396 mode=indexing
                n163 = Unbundle By Name(w430) -> ("Name"=w429:string)
              }
              n164 = for {
                tunnel: w399 -> [w418] mode=indexing
                shift-right: [w414] -> w395
                shift-left: i32[] [] -> [w415]
                tunnel: w396 -> [w412]
                shift-right: [w410] -> _
                shift-left: w400 -> [w411]
                n165 = Unbundle By Name(w418) -> ("Name"=w417:string)
                n166 = call "CRYFind Same Name.vi"("Name"=w417, "sNames"=w411) -> ("bResult"=w416:bool, "NameOut"=w413:string)  [unwired: 7 in, 1 out]
                n167 = case shown="True" w416 {
                  tunnel: w415 -> [w420 w428]
                  tunnel: [w420 w427] -> w414
                  tunnel: w413 -> [_ w422]
                  tunnel: w412 -> [_ w426]
                  tunnel: w411 -> [w419 w423]
                  tunnel: [w419 w424] -> w410
                  frame False {
                  }
                  frame True {
                    n168 = Search 1D Array(1D array=w426, element=w422) -> (index of element=w425:i32)  [unwired: 1 in]
                    n169 = Search 1D Array(1D array=w423, element=w422) -> (index of element=w421:i32)  [unwired: 1 in]
                    n170 = Delete From Array(array=w423, index=w421) -> (array with subset deleted=w424:string[])  [unwired: 1 in, 1 out]
                    n171 = Insert Into Array(array=w428, new element=w425) -> (w427:i32[])  [unwired: 1 in]
                  }
                }
              }
              "wav1" <- w395
              n172 = call "CRYInsert Waveform.vi"("sOptionUpdate"="Run", "Index"=w394, "Waveform"=w399) -> ("Inserted Index"=w408:i32[], "Inserted Name Out"=w409:string[])  [unwired: 1 in, 6 out]
            }
          }
        }
      }
    }
    frame "Overwrite" {
      n173 = flat-sequence {
        tunnel: [w467] -> w445
        frame #0 {
          w467 = TRUE ("OverwriteStart")
          n174 = global write "CRYCurve Library Global.vi" "OverwriteNumber"(-1 ("OverwriteNumber")) -> ()
          n175 = global write "CRYCurve Library Global.vi" "OverwriteStart"(w467) -> ()
        }
      }
      n176 = Equal?(x=w444, y=-100) -> (x = y?=w447:bool)
      n177 = Select(t="CalibrateOverwrite_NoCalSignal" ("f"), s=w447, f="") -> (s? t:f=w446:string)
      n178 = case shown="\"Curves\", \"Values\", Default" w463 {
        tunnel: w465 -> [w469 _ _]
        tunnel: [w472 w480 w488] -> w459
        tunnel: [w471 w479 w487] -> w458
        tunnel: w453 -> [_ w477 _]
        tunnel: w452 -> [_ _ w485]
        tunnel: [w468 w476 w484] -> w451
        tunnel: w445 -> [_ _ _]
        frame "Curves", "Values", Default {
          n179 = for {
            tunnel: w469 -> [w473] mode=indexing
            tunnel: [w475] -> w472 mode=indexing
            tunnel: [w474] -> w471 mode=indexing
            n180 = Unbundle By Name(w473) -> ("Name"=w475:string, "Step No."=w474:i32)
          }
          n181 = Array Size(array=w469) -> (size(s)=w470:i32)
          n182 = Decrement(x=w470) -> (x-1=w468:i32)
        }
        frame "Results" {
          n183 = for {
            tunnel: w477 -> [w481] mode=indexing
            tunnel: [w483] -> w480 mode=indexing
            tunnel: [w482] -> w479 mode=indexing
            n184 = Unbundle By Name(w481) -> ("Name"=w483:string, "Step No."=w482:i32)
          }
          n185 = Array Size(array=w477) -> (size(s)=w478:i32)
          n186 = Decrement(x=w478) -> (x-1=w476:i32)
        }
        frame "WFM" {
          n187 = for {
            tunnel: w485 -> [w489] mode=indexing
            tunnel: [w491] -> w488 mode=indexing
            tunnel: [w490] -> w487 mode=indexing
            n188 = Unbundle By Name(w489) -> ("Name"=w491:string, "Step No."=w490:i32)
          }
          n189 = Array Size(array=w485) -> (size(s)=w486:i32)
          n190 = Decrement(x=w486) -> (x-1=w484:i32)
        }
      }
      n191 = for {
        shift-right: [w502] -> _
        shift-left: -1 ("Inserted index") -> [w503]
        tunnel: w463 -> [w508]
        tunnel: [w500] -> w462
        tunnel: w451 -> [w506]
        tunnel: w459 -> [w504]
        tunnel: w463 -> [w495]
        tunnel: w459 -> [w499] mode=indexing
        tunnel: w458 -> [w500] mode=indexing
        tunnel: w446 -> [w494]
        i -> [w496]
        n192 = flat-sequence {
          tunnel: [w515] -> w492
          frame #0 {
            w515 = "" ("OverwriteStatus")
            n193 = global write "CRYCurve Library Global.vi" "OverwriteStatus"(w515) -> ()
          }
        }
        n194 = Equal?(x=w506, y=w496) -> (x = y?=w505:bool)
        n195 = call "CRYGet Curve Library Data Name.vi"("sAction"="All") -> ("nStep No"=w509:i32[], "sNames"=w497:string[])  [unwired: 7 in, 2 out]
        n196 = Search 1D Array(1D array=w497, element=w499) -> (index of element=w513:i32)  [unwired: 1 in]
        n197 = case shown="-1" w513 {
          selector: w513 -> [_ w660]
          tunnel: w500 -> [w602 w669]
          tunnel: w499 -> [w601 w668]
          tunnel: [w600 w674] -> w510
          tunnel: w503 -> [w598 w667]
          tunnel: [w597 w673] -> w512
          tunnel: [w596 w671] -> w511
          tunnel: w509 -> [_ w672]
          tunnel: w508 -> [w594 w662]
          tunnel: w505 -> [w593 w665]
          tunnel: w504 -> [w591 w664]
          tunnel: w496 -> [w590 w663]
          tunnel: w495 -> [w589 _]
          tunnel: [_ w658] -> w498
          tunnel: w497 -> [_ w661]
          tunnel: w492 -> [_ _]
          frame -1 {
            n198 = Build Array(w602) -> (w603:i32[])
            n199 = call "CRYGet Curve Library Data Name.vi"("nData"=w603, "sOption"="byType", "sAction"="GetNamebyStep", "Type"=w594) -> ("sNames"=w599:string[])  [unwired: 4 in, 3 out]
            n200 = Array Size(array=w599) -> (size(s)=w592:i32)
            n201 = case shown="Default" w592 {
              tunnel: w601 -> [w616 _]
              tunnel: [w615 "FlagAppend" ("sAction")] -> w600
              tunnel: w599 -> [w605 _]
              tunnel: w598 -> [w614 _]
              tunnel: [w612 "Insert" ("sAction")] -> w597
              tunnel: [w611 -1 ("Index")] -> w596
              tunnel: w593 -> [w609 _]
              tunnel: w591 -> [w608 _]
              tunnel: w590 -> [w607 _]
              tunnel: w589 -> [w606 _]
              frame Default {
                n202 = call "CRYFind Same Name.vi"("Name"=w616, "sNames"=w605) -> ("bResult"=w610:bool, "Index"=w613:i32)  [unwired: 7 in, 1 out]
                n203 = case shown="False" w610 {
                  tunnel: ["FlagAppend" ("sAction") "FlagAppend" ("sAction")] -> w615
                  tunnel: w614 -> [w625 _]
                  tunnel: w613 -> [_ w652]
                  tunnel: ["Insert" ("sAction") "Replace_KeepName" ("sAction")] -> w612
                  tunnel: [w622 w652] -> w611
                  tunnel: w609 -> [w621 _]
                  tunnel: w605 -> [w620 _]
                  tunnel: w608 -> [w619 _]
                  tunnel: w607 -> [w618 _]
                  tunnel: w606 -> [w617 _]
                  frame False {
                    n204 = Equal?(x=w625, y=-1) -> (x = y?=w623:bool)
                    n205 = case shown="True" w623 {
                      tunnel: w625 -> [w629 _]
                      tunnel: [w628 w634] -> w622
                      tunnel: w621 -> [_ w635]
                      tunnel: w620 -> [_ w633]
                      tunnel: w619 -> [_ w632]
                      tunnel: w618 -> [_ w631]
                      tunnel: w617 -> [_ w630]
                      frame False {
                        n206 = Increment(x=w629) -> (x+1=w628:i32)
                      }
                      frame True {
                        n207 = case shown="False" w635 {
                          tunnel: [w641 -1] -> w634
                          tunnel: w633 -> [w646 _]
                          tunnel: w632 -> [w645 _]
                          tunnel: w631 -> [w644 _]
                          tunnel: w630 -> [w636 _]
                          frame False {
                            n208 = Increment(x=w644) -> (x+1=w642:i32)
                            n209 = Array Subset(array=w645, index=w642) -> (w643:string[])  [unwired: 1 in]
                            n210 = for {
                              tunnel: w646 -> [w650]
                              tunnel: [w649] -> w640
                              tunnel: w643 -> [w648] mode=indexing
                              tunnel: [w647] -> w638
                              stop <- w649 stop-if-true
                              n211 = call "CRYFind Same Name.vi"("Name"=w648, "sNames"=w650) -> ("bResult"=w649:bool, "NameOut"=w647:string)  [unwired: 7 in, 1 out]
                            }
                            n212 = call "CRYGet Curve Library Data.vi"("Type"=w636, "Data Name"=w638) -> ("index"=w637:i32)  [unwired: 4 out]
                            n213 = Select(t=w637, s=w640, f=-1 ("y")) -> (s? t:f=w641:i32)
                          }
                          frame True {
                          }
                        }
                      }
                    }
                  }
                  frame True {
                  }
                }
              }
              frame 0 {
              }
            }
          }
          frame 0, Default {
            n214 = Index Array(array=w672, index=w660) -> (element=w666:i32)
            n215 = Index Array(array=w661, index=w660) -> (element=w659:string)
            n216 = Equal?(x=w662, y=w666) -> (x = y?=w670:bool)
            n217 = case shown="True" w670 {
              tunnel: ["FlagAppend" ("sAction") w730] -> w674
              tunnel: ["Insert" ("sAction") "Replace_KeepStepNo" ("sAction")] -> w673
              tunnel: [w680 w724] -> w671
              tunnel: w660 -> [_ _]
              tunnel: w669 -> [w685 w726]
              tunnel: w668 -> [_ w727]
              tunnel: w667 -> [w684 _]
              tunnel: w666 -> [w677 w725]
              tunnel: w665 -> [w683 _]
              tunnel: w664 -> [w682 _]
              tunnel: w663 -> [w681 _]
              tunnel: w662 -> [w678 _]
              tunnel: [_ w722] -> w658
              tunnel: w659 -> [w679 _]
              frame False {
                n218 = call "CRYGet Curve Library Data.vi"("Type"=w677, "Data Name"=w679) -> ("index"=w676:i32)  [unwired: 4 out]
                n219 = Build Array(w685) -> (w689:i32[])
                n220 = Build Array(w676) -> (w675:i32[])
                n221 = call "CRYGet Curve Library Data Name.vi"("nData"=w689, "sOption"="byType", "sAction"="GetNamebyStep", "Type"=w678) -> ("sNames"=w691:string[])  [unwired: 4 in, 3 out]
                n222 = Equal?(x=w684, y=-1) -> (x = y?=w686:bool)
                n223 = case shown="True" w686 {
                  tunnel: w684 -> [w699 _]
                  tunnel: [w698 w704] -> w680
                  tunnel: w683 -> [_ w705]
                  tunnel: w691 -> [_ w703]
                  tunnel: w682 -> [_ w702]
                  tunnel: w681 -> [_ w701]
                  tunnel: w678 -> [_ w700]
                  frame False {
                    n224 = Increment(x=w699) -> (x+1=w698:i32)
                  }
                  frame True {
                    n225 = case shown="False" w705 {
                      tunnel: [w711 -1] -> w704
                      tunnel: w703 -> [w716 _]
                      tunnel: w702 -> [w715 _]
                      tunnel: w701 -> [w714 _]
                      tunnel: w700 -> [w706 _]
                      frame False {
                        n226 = Increment(x=w714) -> (x+1=w712:i32)
                        n227 = Array Subset(array=w715, index=w712) -> (w713:string[])  [unwired: 1 in]
                        n228 = for {
                          tunnel: w716 -> [w720]
                          tunnel: [w719] -> w710
                          tunnel: w713 -> [w718] mode=indexing
                          tunnel: [w717] -> w708
                          stop <- w719 stop-if-true
                          n229 = call "CRYFind Same Name.vi"("Name"=w718, "sNames"=w720) -> ("bResult"=w719:bool, "NameOut"=w717:string)  [unwired: 7 in, 1 out]
                        }
                        n230 = call "CRYGet Curve Library Data.vi"("Type"=w706, "Data Name"=w708) -> ("index"=w707:i32)  [unwired: 4 out]
                        n231 = Select(t=w707, s=w710, f=-1 ("y")) -> (s? t:f=w711:i32)
                      }
                      frame True {
                      }
                    }
                  }
                }
                n232 = call "CRYChange Curve Library.vi"("Index"=w675, "Type In"=w677, "sAction"="Delete") -> ("Name Out"=w692:string[])  [unwired: 7 in, 1 out]
                n233 = local read "Deleted Names"() -> (w694:string[])
                n234 = Insert Into Array(array=w694, new element=w692) -> (w693:string[])  [unwired: 1 in]
                n235 = local write "Deleted Names"(w693) -> ()
              }
              frame True {
                n236 = call "CRYGet Curve Library Data.vi"("Type"=w725, "Data Name"=w727) -> ("Step No."=w723:i32, "index"=w724:i32)  [unwired: 3 out]
                n237 = Equal?(x=w723, y=w726) -> (x = y?=w728:bool)
                n238 = case shown="False" w728 {
                  tunnel: ["FlagAppend" ("sAction") w732] -> w730
                  tunnel: w723 -> [_ w734]
                  tunnel: [_ w739] -> w722
                  frame True {
                  }
                  frame False {
                    w732 = "StepNo_NotEqual" ("sAction")
                    n239 = Number To Decimal String(number=w734) -> (decimal integer string=w735:string)  [unwired: 1 in]
                    n240 = Concatenate Strings("CalibrateOverwrite" ("f"), "#" ("string"), w735) -> (w733:string)
                    n241 = global write "CRYCurve Library Global.vi" "OverwriteStatus"(w732) -> ()
                    n242 = call "CRYCheck Calibration Step.vi"("Step No"=w734) -> ("Is Calibration?"=w738:bool)  [unwired: 9 in, 1 out]
                    n243 = Select(t=w733, s=w738, f="") -> (s? t:f=w739:string)
                  }
                }
              }
            }
          }
        }
        n244 = case shown="\"Insert\", \"Replace_KeepName\", \"Replace_KeepStepNo\"" w512 {
          selector: w512 -> [w551 w587]
          tunnel: [w547 i32[] [] ("Inserted index")] -> w501
          tunnel: w511 -> [w552 _]
          tunnel: w510 -> [w548 _]
          tunnel: [w548 "Nothing" ("sAction")] -> w493
          tunnel: w495 -> [w541 _]
          tunnel: [w551 w587] -> w507
          tunnel: w498 -> [w544 _]
          tunnel: w494 -> [w543 _]
          tunnel: w496 -> [w542 _]
          frame "Insert", "Replace_KeepName", "Replace_KeepStepNo" {
            n245 = case shown="\"Curves\", \"Values\", Default" w541 {
              selector: w541 -> [w557 w568 w579]
              tunnel: w552 -> [w563 w574 w585]
              tunnel: w551 -> [w562 w573 w584]
              tunnel: [w561 w572 w583] -> w540
              tunnel: [w560 w571 w582] -> w547
              tunnel: w544 -> [w559 w570 w581]
              tunnel: w543 -> [w558 w569 w580]
              tunnel: w542 -> [w555 w566 w577]
              frame "Curves", "Values", Default {
                n246 = local read "Curves"() -> (w556:T5)
                n247 = Build Array(w563) -> (w553:i32[])
                n248 = Index Array(array=w556, index=w555) -> (element=w554:T6)
                n249 = call "CRYChange Curve Library.vi"("sOptioin 2"=w558, "sOptioin 1"=w559, "Index"=w553, "Curve"=w554, "Type In"=w557, "sAction"=w562) -> ("Inserted index"=w560:i32[], "Name Out"=w561:string[])  [unwired: 4 in]
              }
              frame "Results" {
                n250 = local read "Results"() -> (w567:T3)
                n251 = Build Array(w574) -> (w564:i32[])
                n252 = Index Array(array=w567, index=w566) -> (element=w565:T4)
                n253 = call "CRYChange Curve Library.vi"("sOptioin 2"=w569, "Result"=w565, "sOptioin 1"=w570, "Index"=w564, "Type In"=w568, "sAction"=w573) -> ("Inserted index"=w571:i32[], "Name Out"=w572:string[])  [unwired: 4 in]
              }
              frame "WFM" {
                n254 = local read "Waves"() -> (w578:T1)
                n255 = Build Array(w585) -> (w575:i32[])
                n256 = Index Array(array=w578, index=w577) -> (element=w576:T2)
                n257 = call "CRYChange Curve Library.vi"("Waveform"=w576, "sOptioin 2"=w580, "sOptioin 1"=w581, "Index"=w575, "Type In"=w579, "sAction"=w584) -> ("Inserted index"=w582:i32[], "Name Out"=w583:string[])  [unwired: 4 in]
              }
            }
            n258 = local read "Inserted Names"() -> (w549:string[])
            n259 = local read "Inserted Index"() -> (w546:i32[])
            n260 = Insert Into Array(array=w546, new element=w547) -> (w545:i32[])  [unwired: 1 in]
            n261 = local write "Inserted Index"(w545) -> ()
            n262 = Insert Into Array(array=w549, new element=w540) -> (w550:string[])  [unwired: 1 in]
            n263 = local write "Inserted Names"(w550) -> ()
          }
          frame Default {
            # "You cannot come here, this case is invalid"
          }
        }
        n264 = case shown="Default" w493 {
          tunnel: w503 -> [_ w518]
          tunnel: w501 -> [w517 _]
          tunnel: [w516 w518] -> w502
          frame Default {
            n265 = Index Array(array=w517) -> (element=w516:i32)  [unwired: 1 in]
          }
          frame "StepNo_NotEqual" {
          }
        }
        n266 = case shown="Default" w507 {
          tunnel: w493 -> [_ w522]
          tunnel: w495 -> [_ w519]
          tunnel: w500 -> [_ w521]
          tunnel: w499 -> [_ w520]
          frame Default {
          }
          frame "Replace_KeepStepNo" {
            n267 = case shown="\"StepNo_NotEqual\"" w522 {
              tunnel: w521 -> [_ w529]
              tunnel: w520 -> [_ w528]
              tunnel: w519 -> [_ w523]
              frame Default {
              }
              frame "StepNo_NotEqual" {
                n268 = Build Array(w529) -> (w531:i32[])
                n269 = call "CRYGet Curve Library Data Name.vi"("nData"=w531, "sOption"="byType", "sAction"="GetNamebyStep", "Type"=w523) -> ("sNames"=w527:string[])  [unwired: 4 in, 3 out]
                n270 = call "CRYFind Same Name.vi"("Name"=w528, "sNames"=w527) -> ("bResult"=w524:bool, "NameOut"=w526:string)  [unwired: 7 in, 1 out]
                n271 = call "CRYGet Curve Library Data.vi"("Type"=w523, "Data Name"=w526) -> ("index"=w525:i32)  [unwired: 4 out]
                n272 = case shown="True" w524 {
                  tunnel: w523 -> [_ w536]
                  tunnel: w525 -> [_ w535]
                  frame False {
                  }
                  frame True {
                    n273 = local read "Deleted Names"() -> (w539:string[])
                    n274 = Build Array(w535) -> (w533:i32[])
                    n275 = call "CRYChange Curve Library.vi"("Index"=w533, "Type In"=w536, "sAction"="Delete") -> ("Name Out"=w538:string[])  [unwired: 7 in, 1 out]
                    n276 = Insert Into Array(array=w539, new element=w538) -> (w537:string[])  [unwired: 1 in]
                    n277 = local write "Deleted Names"(w537) -> ()
                  }
                }
              }
            }
          }
        }
      }
      n278 = flat-sequence {
        tunnel: w463 -> [w743]
        tunnel: w462 -> [w751]
        tunnel: [w741] -> w457
        tunnel: [w750] -> w456
        tunnel: [w743] -> w455
        tunnel: [w742] -> w454
        tunnel: w446 -> [w749]
        tunnel: [w785] -> w461
        tunnel: [w786] -> w464
        tunnel: w457 -> [w786]
        tunnel: w456 -> [w785]
        tunnel: w455 -> [w784]
        tunnel: w454 -> [w783]
        frame #0 {
          (unwired) "StepNo_NotEqual" ("sAction")
          n279 = local read "Inserted Names"() -> (w741:string[])
          n280 = case shown="Default" w749 {
            tunnel: w751 -> [_ w778]
            tunnel: w743 -> [_ w775]
            tunnel: [string[] [] ("Name Out") w774] -> w742
            tunnel: [i32[] [] ("Inserted Index") w773] -> w750
            frame "CalibrateOverwrite_NoCalSignal" {
            }
            frame Default {
              n281 = local read "Inserted Index"() -> (w773:i32[])
              n282 = Build Array(w778) -> (w780:i32[])
              n283 = call "CRYGet Curve Library Data Name.vi"("nData"=w780, "sOption"="byType", "sAction"="GetNamebyStep", "Type"=w775) -> ("Index"=w777:i32[])  [unwired: 4 in, 3 out]
              n284 = call "CRYGet Difference Array.vi"("Array 2"=w773, "Array 1"=w777) -> ("Diff Out"=w776:i32[])  [unwired: 8 in, 1 out]
              n285 = Sort 1D Array(array=w776) -> (sorted array=w772:i32[])
              n286 = Reverse 1D Array(array=w772) -> (reversed array=w770:i32[])
              n287 = call "CRYChange Curve Library.vi"("Index"=w770, "Type In"=w775, "sAction"="Delete") -> ("Name Out"=w774:string[])  [unwired: 7 in, 1 out]
            }
          }
          n288 = global read "CRYCurve Library Global.vi" "ReplaceNames"() -> (w745:T8)
          n289 = global write "CRYCurve Library Global.vi" "OverwriteStatus"("" ("OverwriteStatus")) -> ()
          n290 = global write "CRYCurve Library Global.vi" "OverwriteNumber"(-1 ("OverwriteNumber")) -> ()
          n291 = global write "CRYCurve Library Global.vi" "OverwriteStart"(FALSE ("OverwriteStart")) -> ()
          n292 = case shown="\"WFM\"" w743 {
            tunnel: w745 -> [w755 w759 w763 w767]
            tunnel: [w754 w758 w762 w766] -> w744
            tunnel: w742 -> [w753 w757 w761 w765]
            tunnel: w741 -> [w752 w756 w760 w764]
            frame "Curves", Default {
              n293 = Bundle By Name(cluster=w755, "CurveOld"=w753, "CurveNew"=w752) -> (w754:T8)
            }
            frame "Values" {
              n294 = Bundle By Name(cluster=w759, "ValueOld"=w757, "ValueNew"=w756) -> (w758:T8)
            }
            frame "Results" {
              n295 = Bundle By Name(cluster=w763, "ResultOld"=w761, "ResultNew"=w760) -> (w762:T8)
            }
            frame "WFM" {
              n296 = Bundle By Name(cluster=w767, "WFMOld"=w765, "WFMNew"=w764) -> (w766:T8)
            }
          }
          n297 = global write "CRYCurve Library Global.vi" "ReplaceNames"(w744) -> ()
        }
        frame #1 {
          n298 = global read "CRYProject Run Control Global.vi" "RunState"() -> (w782:bool)
          n299 = case shown="False" w782 {
            tunnel: w784 -> [w791 _]
            tunnel: w783 -> [w788 _]
            frame False {
              n300 = local read "Deleted Names"() -> (w789:string[])
              n301 = local read "Inserted Names"() -> (w790:string[])
              n302 = local read "Inserted Index"() -> (w792:i32[])
              n303 = Insert Into Array(array=w789, new element=w788) -> (w787:string[])  [unwired: 1 in]
              n304 = call "CRYUpdate Curve Library Graph.vi"("sOption 1"="CurLibGraph" ("sOption"), "Deleted Names"=w787, "Replaced Old Names"=w790, "Index"=w792, "Type"=w791) -> ()  [unwired: 7 in]
            }
            frame True {
            }
          }
        }
      }
    }
  }
  n305 = flat-sequence {
    tunnel: w15 -> [w795]
    frame #0 {
      n306 = global write "CRYCurve Library Global.vi" "Curve Library Global Inserting"(FALSE ("Curve Library Global Inserting")) -> ()
      "Inserted Names Out" <- w795
    }
  }
  "Type Out" <- "Type In"
